vi "Is Safety Button Clicked.vi"(8 "Error In":errorcluster, 11 "device ID":refnum<k1>) -> (0 "Error Out":errorcluster, 3 "device ID":refnum<k1>)   [LabVIEW 2014]
doc: "This VI Informs - is safety button clicked?"
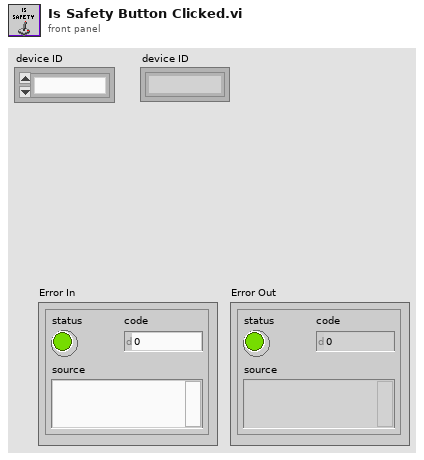
[diagram p1: front panel]
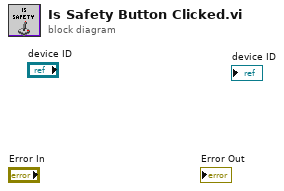
[diagram p0: block diagram]
diagram:
